vi "FEA_Model_Getter.vi"(8 "error in (no error)":errorcluster, 11 "FEA_Model in":refnum<class "FEA_Model.lvclass">) -> (0 "error out":errorcluster, 3 "FEA Model":T1)   [LabVIEW 2021, in "FEA_Model.lvclass"]
uses:
  FEA_Model.lvclass
  FEA_Model.lvclass/FEA_Model.ctl
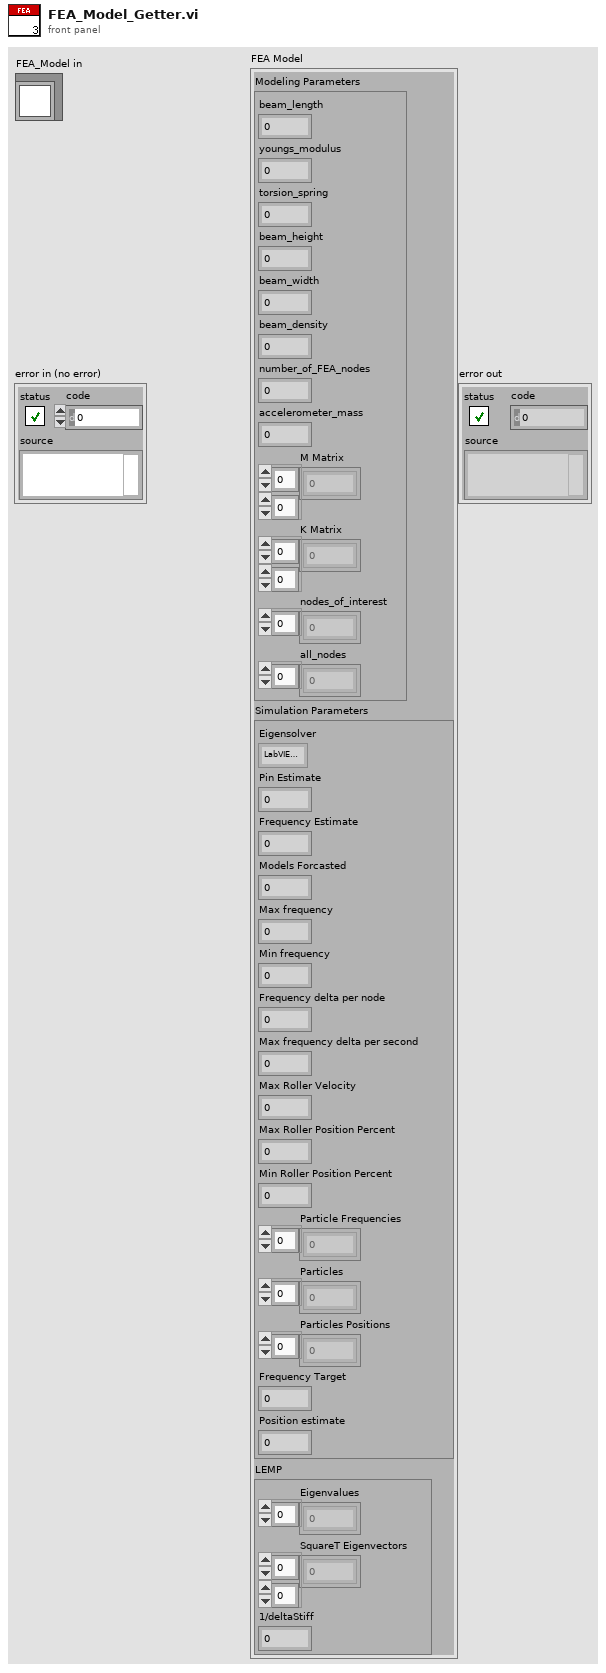
[diagram p1: front panel]
types:
  T1 = cluster{"Modeling Parameters":cluster{"beam_length":dbl, "youngs_modulus":dbl, "torsion_spring":dbl, "beam_height":dbl, "beam_width":dbl, "beam_density":dbl, "number_of_FEA_nodes":i32, "accelerometer_mass":dbl, "M Matrix":dbl[][], "K Matrix":dbl[][], "nodes_of_interest":i32[], "all_nodes":i32[]}, "Simulation Parameters":cluster{"Eigensolver ":enum16{"LabVIEW Cholesky", "LabVIEW General", "LabVIEW Inverse", "LEMP"}, "Pin Estimate":i32, "Frequency Estimate":dbl, "Models Forcasted":i32, "Max frequency":dbl, "Min frequency":dbl, "Frequency delta per node":dbl, "Max frequency delta per second":dbl, "Max Roller Velocity":dbl, "Max Roller Position Percent":dbl, "Min Roller Position Percent":dbl, "Particle Frequencies":dbl[], "Particles":i32[], "Particles Positions":dbl[], "Frequency Target":dbl, "Position estimate":dbl}, "LEMP":cluster{"Eigenvalues":dbl[], "SquareT Eigenvectors":dbl[][], "1/deltaStiff":dbl}}
  T2 = cluster{"beam_length":dbl, "youngs_modulus":dbl, "torsion_spring":dbl, "beam_height":dbl, "beam_width":dbl, "beam_density":dbl, "number_of_FEA_nodes":i32, "accelerometer_mass":dbl, "M Matrix":dbl[][], "K Matrix":dbl[][], "nodes_of_interest":i32[], "all_nodes":i32[]}
  T3 = cluster{"Eigensolver ":enum16{"LabVIEW Cholesky", "LabVIEW General", "LabVIEW Inverse", "LEMP"}, "Pin Estimate":i32, "Frequency Estimate":dbl, "Models Forcasted":i32, "Max frequency":dbl, "Min frequency":dbl, "Frequency delta per node":dbl, "Max frequency delta per second":dbl, "Max Roller Velocity":dbl, "Max Roller Position Percent":dbl, "Min Roller Position Percent":dbl, "Particle Frequencies":dbl[], "Particles":i32[], "Particles Positions":dbl[], "Frequency Target":dbl, "Position estimate":dbl}
  T4 = cluster{"Eigenvalues":dbl[], "SquareT Eigenvectors":dbl[][], "1/deltaStiff":dbl}
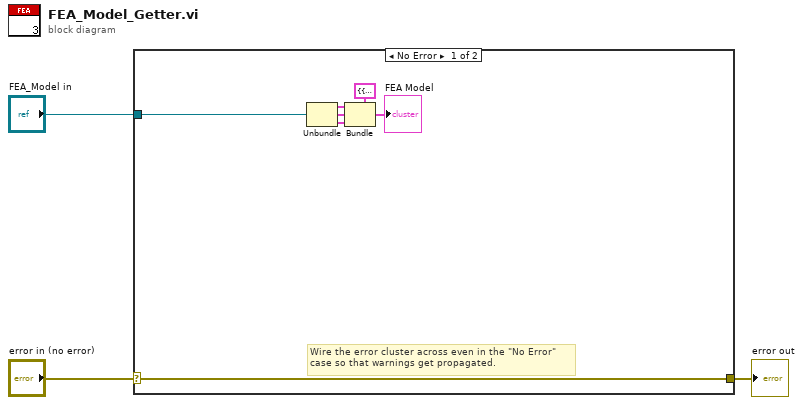
[diagram p0: block diagram]
diagram:
  n1 = case shown="No Error" "error in (no error)" {
    selector: "error in (no error)" -> [w10 w11]
    tunnel: [w10 w11] -> w2
    tunnel: "FEA_Model in" -> [w7 _]
    frame No Error {
      # "Wire the error cluster across even in the \"No Error\"\ncase so that warnings get propagated."
      n2 = Unbundle(w7) -> (w6:T2, w5:T3, w4:T4)
      n3 = Bundle(cluster=T1 {"Modeling Parameters"={"beam_length"=0.0, "youngs_modulus"=0.0, "torsion_spring"=0.0, "beam_height"=0.0, "beam_width"=0.0, "beam_density"=0.0, "number_of_FEA_nodes"=0, "accelerometer_mass"=0.0, "M Matrix"=[], "K Matrix"=[], "nodes_of_interest"=[], "all_nodes"=[]}, "Simulation Parameters"={"Eigensolver "=enum."LabVIEW Cholesky", "Pin Estimate"=0, "Frequency Estimate"=0.0, "Models Forcasted"=0, "Max frequency"=0.0, "Min frequency"=0.0, "Frequency delta per node"=0.0, "Max frequency delta per second"=0.0, "Max Roller Velocity"=0.0, "Max Roller Position Percent"=0.0, "Min Roller Position Percent"=0.0, "Particle Frequencies"=[], "Particles"=[], "Particles Positions"=[], "Frequency Target"=0.0, "Position estimate"=0.0}, "LEMP"={"Eigenvalues"=[], "SquareT Eigenvectors"=[], "1/deltaStiff"=0.0}}, "Modeling Parameters"=w6, "Simulation Parameters"=w5, "LEMP"=w4) -> (→"FEA Model":T1)
    }
    frame Error {
    }
  }
  "error out" <- w2
